vi "parse_formula.vi"(2 "Vi":dbl[](array[numeric])=[1.0, 5.0, 3.9968028886505635e-15, 3.9968028886505635e-15, 3.9968028886505635e-15, 14.693877551020412] format="%#.6f", 3 "formula":string="r=(v2,v3,v4) s=(10,10,10)") -> (1 "result matrix":dbl[][](array[numeric])=[[10.0, -6.975736996017264e-16, -6.975736996017264e-16, 0.0], [6.975736996017264e-16, 10.0, -6.975736996017264e-16, 0.0], [6.975736996017264e-16, 6.975736996017264e-16, 10.0, 0.0], [0.0, 0.0, 0.0, 1.0]] format="%#.6f")   [LabVIEW 2011]
uses:
  <vilib>/Analysis/baseanly.llb/Real A x B.vi
  <vilib>/Analysis/NI_AALBase.lvlib
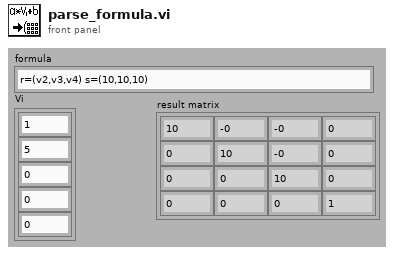
[diagram p1: front panel]
types:
  T1 = typedef "NI_Matrix.lvlib/RealMatrix.ctl" = dbl[][]
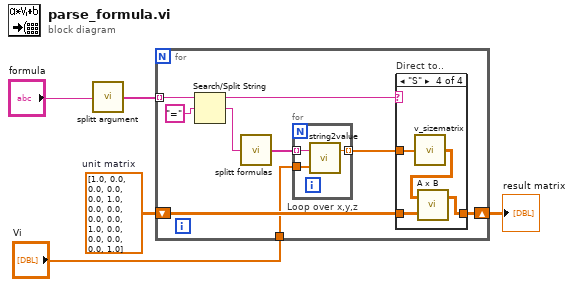
[diagram p0: block diagram]
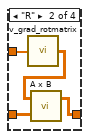
[diagram p3: hidden frame]
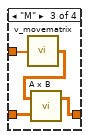
[diagram p4: hidden frame]
diagram:
  w3 = dbl[][] [[1.0, 0.0, 0.0, 0.0], [0.0, 1.0, 0.0, 0.0], [0.0, 0.0, 1.0, 0.0], [0.0, 0.0, 0.0, 1.0]]  # unit matrix
  n1 = call "splitt argument.vi"("formula"="formula") -> ("Array"=w5:string[])
  n2 = for {
    tunnel: w5 -> [w14] mode=indexing
    tunnel: "Vi" -> [w7]
    shift-right: [w10] -> w2
    shift-left: w3 -> [w11]
    n3 = Search/Split String(string=w14, search string/char (-)="=") -> (substring before match=w9:string, match + rest of string=w12:string)  [unwired: 1 in, 1 out]
    n4 = call "splitt formulas.vi"("formula"=w12) -> ("Array"=w8:string[])
    n5 = for "Loop over x,y,z" {
      tunnel: w8 -> [w17] mode=indexing
      tunnel: w7 -> [w16]
      tunnel: [w15] -> w6 mode=indexing
      n6 = call "string2value.vi"("variables"=w16, "String"=w17) -> ("value"=w15:dbl)  [unwired: 1 in]
    }
    n7 = case "Direct to.." shown="\"S\"" w9 {
      tunnel: w11 -> [w18 w22 w25 w29]
      tunnel: [w18 w21 w24 w28] -> w10
      tunnel: w6 -> [_ w19 w23 w27]
      frame "False", Default {
      }
      frame "R" {
        n8 = call "v_grad_rotmatrix.vi"("grad_xyz"=w19) -> ("rotate matrix"=w20:dbl[][])
        n9 = call-poly <vilib>:"A x B.vi"("B"=w22, "A"=w20) -> ("A x B"=w21:T1)  [unwired: 1 out]
      }
      frame "M" {
        n10 = call "v_movematrix.vi"("xyz"=w23) -> ("matrix"=w26:dbl[][])
        n11 = call-poly <vilib>:"A x B.vi"("B"=w25, "A"=w26) -> ("A x B"=w24:T1)  [unwired: 1 out]
      }
      frame "S" {
        n12 = call "v_sizematrix.vi"("xyz"=w27) -> ("matrix"=w30:dbl[][])
        n13 = call-poly <vilib>:"A x B.vi"("B"=w29, "A"=w30) -> ("A x B"=w28:T1)  [unwired: 1 out]
      }
    }
  }
  "result matrix" <- w2
